vi "N5765A_ReadCurrent.vi"(8 "error in (no error)":errorcluster, 11 "VISA resource name":refnum<visa-resource-name>="PS2") -> (0 "error out":errorcluster, 2 "Measurement":dbl=-0.0009589195 format="%^.3e", 3 "VISA out":refnum<visa-resource-name>)   [LabVIEW 2015]
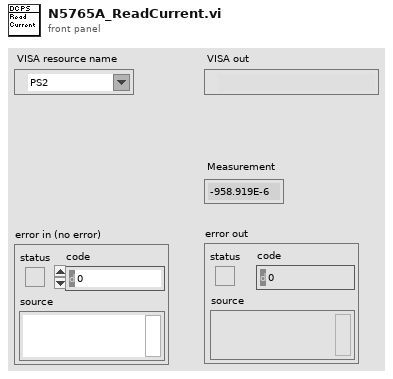
[diagram p1: front panel]
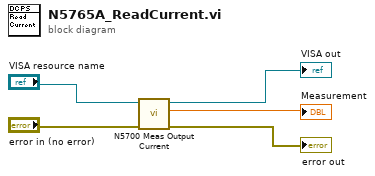
[diagram p0: block diagram]
diagram:
  n1 = call <instrlib>:"N5700 Meas Output Current.vi"("error"="error in (no error)", "VISA"="VISA resource name") -> ("error out"=→"error out":errorcluster, "Output Current"=→"Measurement":dbl, "VISA out"=→"VISA out":refnum<visa-resource-name>)  [unwired: 4 in]
